vi "Rcv Cmd.vi"(8 "error in":errorcluster, 11 "Instrument in":refnum<class "Instrument.lvclass">) -> (0 "error out":errorcluster, 3 "Instrument out":refnum<class "Instrument.lvclass">)   [LabVIEW 2015, in "Instrument.lvclass"]
doc: "The Wait method provides a way of defining interaction with the Instrument object during idle times. The default behavior is to listen to the command queue for incoming commands."
uses:
  Instrument.lvclass
  Instrument.lvclass/Instrument.ctl
  Commands/Command.lvclass
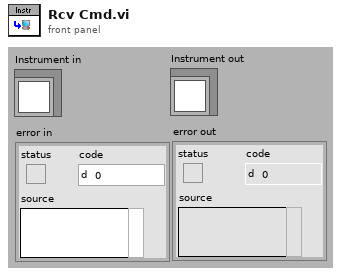
[diagram p1: front panel]
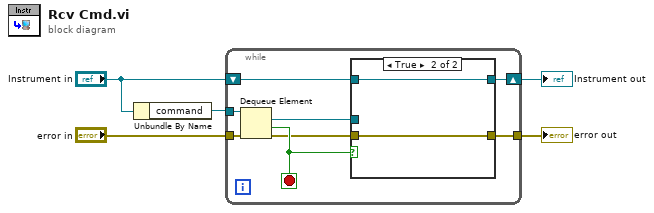
[diagram p0: block diagram]
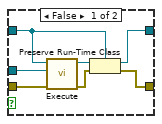
[diagram p2: hidden frame]
diagram:
  n1 = Unbundle By Name("Instrument in") -> ("command"=w1:refnum<queue>)
  n2 = while {
    shift-right: [w12] -> w2
    shift-left: "Instrument in" -> [w13]
    tunnel: w1 -> [w11]
    tunnel: "error in" -> [w8]
    tunnel: [w6] -> w4
    stop <- w10 stop-if-true
    n3 = Dequeue Element(queue=w11, error in (no error)=w8) -> (element=w9:refnum<class "Command.lvclass">, timed out?=w10:bool, error out=w7:errorcluster)  [unwired: 1 in, 1 out]
    n4 = case shown="True" w10 {
      tunnel: w13 -> [w19 w22]
      tunnel: [w18 w22] -> w12
      tunnel: w9 -> [w17 _]
      tunnel: w7 -> [w16 w21]
      tunnel: [w14 w21] -> w6
      frame False {
        n5 = call-dynamic "Execute.vi"("error in"=w16, "Command in"=w17, "Instrument In"=w19) -> ("error out"=w15:errorcluster, "Instrument Out"=w20:refnum<class>)  [unwired: 7 in]
        n6 = Preserve Run-Time Class(object in=w20, error in=w15, 2:w19) -> (object out=w18:refnum<class "Instrument.lvclass">, error out=w14:errorcluster)
      }
      frame True {
      }
    }
  }
  "error out" <- w4
  "Instrument out" <- w2
